vi "读取-缓存数据文件夹至报警记录列表-网络版.vi"() -> (0 "文件名":string[](array[string]), 1 "新记录文件名":string[](array[string]), 2 "新记录列表":string[][](array[string]), 3 "报警记录列表":string[][](array[string]))   [LabVIEW 2017]
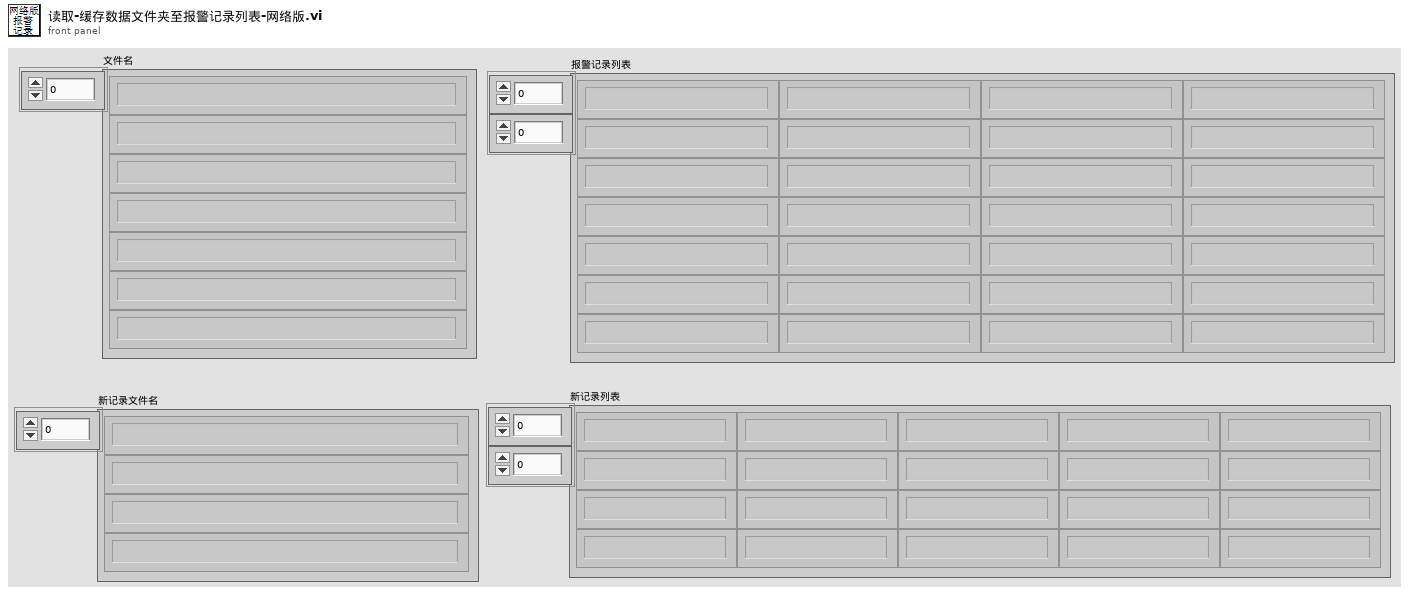
[diagram p1: front panel]
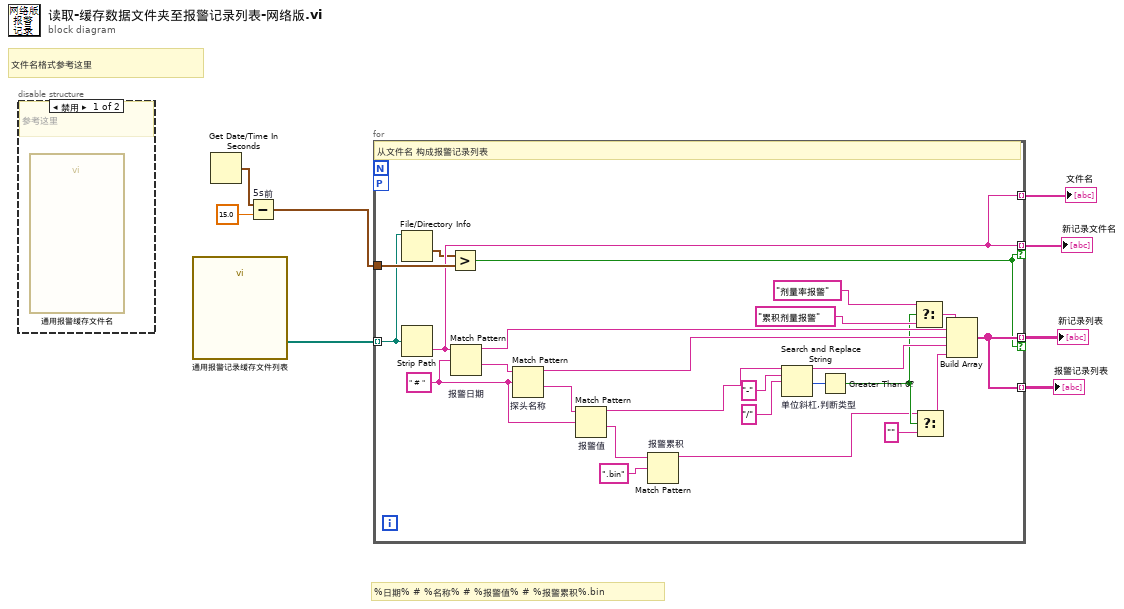
[diagram p0: block diagram]
diagram:
  # "%日期% # %名称% # %报警值% # %报警累积%.bin"
  # "文件名格式参考这里"
  n1 = disable-structure shown="禁用" {
    frame Disabled {
      # "参考这里"
      n2 = call "通用报警缓存文件名.vi"() -> ()  [unwired: 11 in, 1 out]
    }
    frame Enabled {
    }
  }
  n3 = call "通用报警记录缓存文件列表.vi"() -> ("报警记录文件"=w3:path[])  [unwired: 11 in]
  n4 = Get Date/Time In Seconds() -> (seconds since 1Jan1904=w6:timestamp)
  n5 = Subtract "5s前"(x=w6, y=15.0) -> (x-y=w1:timestamp)
  n6 = for "For循环" {
    workers-P: _ -> [_]
    tunnel: [w30] -> w8 mode=indexing
    tunnel: w1 -> [w31]
    tunnel: [w30] -> w5 mode=indexing if=w29
    tunnel: [w27] -> w4 mode=indexing if=w29
    tunnel: w3 -> [w28] mode=indexing
    tunnel: [w27] -> w2 mode=indexing
    w14 = " # " ("正则表达式")
    # "从文件名 构成报警记录列表"
    n7 = File/Directory Info(path=w28) -> (last mod=w26:timestamp)  [unwired: 1 in, 6 out]
    n8 = Strip Path(path=w28) -> (name=w27:string)  [unwired: 1 out]
    n9 = Greater?(x=w26, y=w31) -> (0:w29:bool)
    n10 = Match Pattern "报警日期"(string=w27, regular expression=w14) -> (before substring=w25:string, after substring=w33:string)  [unwired: 1 in, 2 out]
    n11 = Match Pattern "探头名称"(string=w33, regular expression=w14) -> (before substring=w32:string, after substring=w13:string)  [unwired: 1 in, 2 out]
    n12 = Match Pattern "报警值"(string=w13, regular expression=w14) -> (before substring=w10:string, after substring=w11:string)  [unwired: 1 in, 2 out]
    n13 = Match Pattern "报警累积"(string=w11, regular expression=".bin" ("正则表达式")) -> (before substring=w9:string)  [unwired: 1 in, 3 out]
    n14 = Search and Replace String "单位斜杠,判断类型"(input string=w10, search string="-" ("搜索字符串"), replace string="/" ("搜索字符串")) -> (result string=w24:string, number of replacements=w21:i32)  [unwired: 5 in, 2 out]
    n15 = Greater Than 0?(x=w21) -> (x > 0?=w17:bool)
    n16 = Select(t="剂量率报警" ("正则表达式"), s=w17, f="累积剂量报警" ("正则表达式")) -> (s? t:f=w18:string)
    n17 = Select(t=w9, s=w17, f="" ("正则表达式")) -> (s? t:f=w15:string)
    n18 = Build Array(w18, w25, w32, w24, w15) -> (w30:string[])
  }
  "文件名" <- w2
  "报警记录列表" <- w8
  "新记录列表" <- w5
  "新记录文件名" <- w4
